vi "Signals.Scale.Raw.vi"(6 "Type":T1, 7 "Lookup":variant, 8 "error in":errorcluster, 10 "ID":u32, 11 "Writes Ref":T2) -> (0 "error out":errorcluster, 2 "Data":u8[](array[numeric]))   [LabVIEW 2019, in "Diagnostics Addon Engine.lvlib"]
uses:
  Diagnostics Addon Engine.lvlib
  <vilib>/NI/NIVS Inline Async API/_Data Access Engine/Data Access Engine/Types/Read.DVR.ctl
  <vilib>/NI/NIVS Inline Async API/_Data Access Engine/Access Type Classes/Read/Read.lvclass
  Shared/Types/Type.ctl
  Shared/Types/Frame.Lookup.Info.ctl
  <vilib>/NI/NIVS Inline Async API/_Data Access Engine/Access Type Classes/Read/Read.lvclass/Read.ctl
  <vilib>/NI/NIVS Inline Async API/_Data Access Engine/Data Access Engine/Methods/Read.Data.vi
  <vilib>/NI/NIVS Inline Async API/_Data Access Engine/Access Type Classes/Read/Read.ProcessData.vi
  Shared/SubVIs/Constants.vi
  <vilib>/xnet/xnet.llb/XNET Convert (Signal to Frame CAN).vi
  Shared/Diagnostics Addon Shared.lvlib
  <vilib>/NI VeriStand/Custom Device Tools/Custom Device Utility Library/Custom Device Utility Library.lvlib
  <vilib>/NI/NIVS Inline Async API/_Data Access Engine/Data Access Engine/Data Access Engine.lvclass
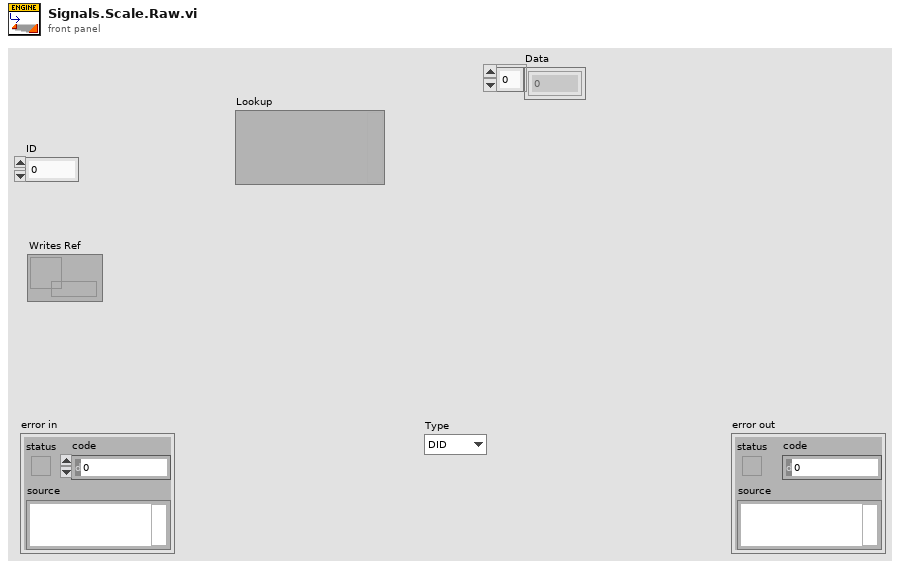
[diagram p1: front panel]
types:
  T1 = typedef "Diagnostics Addon Shared.lvlib/Type.ctl" = enum16{"DID", "CDID", "PID", "CPID", "Read Memory", "Write Memory", "DTC Control", "IO Cmd", "IO Resp", "Routine Start Cmd", "Routine Start Resp", "Routine Request Cmd", "Routine Request Resp", "Routine Stop Cmd", "Routine Stop Resp", "UserDefined Cmd", "UserDefined Rsp"}
  T2 = typedef "Data Access Engine.lvlib/Data Access Engine.lvclass/Read.DVR.ctl" = refnum<data-value>
  T3 = typedef "Diagnostics Addon Shared.lvlib/Frame.Lookup.Info.ctl" = cluster{"Offset":i32, "Length":i32, "ByteLength":u16}
  T4 = typedef "XNET Frame CAN.ctl" = cluster{"timestamp":timestamp, "payload":u8[], "identifier":u32, "type":T5, "extended?":bool, "echo?":bool}
  T5 = typedef "XNET Frame Type CAN.ctl" = u8
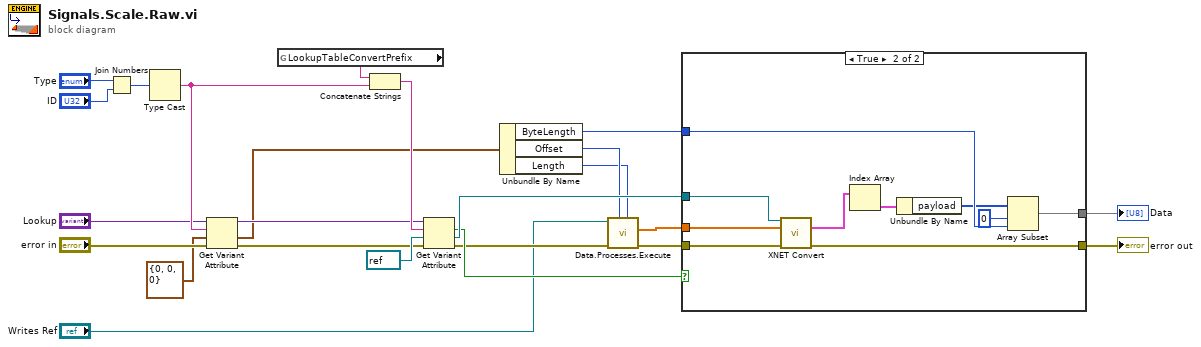
[diagram p0: block diagram]
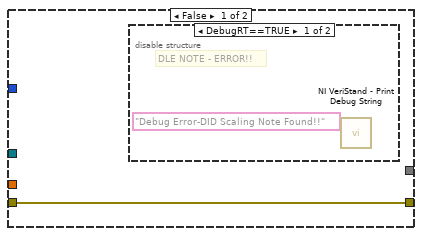
[diagram p2: hidden frame]
diagram:
  n1 = Join Numbers(hi="Type", lo="ID") -> ((hi.lo)=w8:u64)
  n2 = Type Cast(x=w8) -> (*(type *) &x=w18:string)  [unwired: 1 in]
  n3 = Get Variant Attribute(Variant="Lookup", name=w18, default value (empty Variant)=T3 {"Offset"=0, "Length"=0, "ByteLength"=0} ("cluster"), error in="error in") -> (duplicate Variant=w17:variant, value=w12:T3, error out=w19:errorcluster)  [unwired: 1 out]
  n4 = global read "Constants.vi" "LookupTableConvertPrefix"() -> (w20:string)
  n5 = Concatenate Strings(w20, w18) -> (w21:string)
  n6 = Get Variant Attribute(Variant=w17, name=w21, default value (empty Variant)=refnum<k21> refnum ("DID Conversion"), error in=w19) -> (found=w7:bool, value=w13:refnum<k21>, error out=w3:errorcluster)  [unwired: 1 out]
  n7 = Unbundle By Name(w12) -> ("ByteLength"=w15:u16, "Offset"=w6:i32, "Length"=w5:i32)
  n8 = call-poly <vilib>:"Data.Processes.Execute.vi"("length"=w5, "index"=w6, "error in (no error)"=w3, "Ref"="Writes Ref") -> ("error out"=w2:errorcluster, "Values"=w4:dbl[])  [unwired: 5 in, 1 out]
  n9 = case shown="True" w7 {
    tunnel: w2 -> [w25 w36]
    tunnel: [w25 w30] -> w11
    tunnel: w4 -> [_ w32]
    tunnel: w13 -> [_ w35]
    tunnel: w15 -> [_ w33]
    tunnel: [_ w31] -> w14
    frame False {
      n10 = disable-structure shown="DebugRT==TRUE" {
        frame condition #0 {
          # "DLE NOTE - ERROR!!"
          n11 = call <vilib>:"NI VeriStand - Print Debug String.vi"("Message"="Debug Error-DID Scaling Note Found!!" ("Debug String")) -> ()  [unwired: 10 in, 1 out]
        }
        frame condition #1 (active) {
        }
      }
    }
    frame True {
      n12 = call-poly <vilib>:"XNET Convert.vi"("session in"=w35, "signal data"=w32, "error in (no error)"=w36) -> ("frame data"=w29:T4[], "error out"=w30:errorcluster)  [unwired: 9 in, 2 out]
      n13 = Index Array(array=w29) -> (element=w28:T4)  [unwired: 1 in]
      n14 = Unbundle By Name(w28) -> ("payload"=w27:u8[])
      n15 = Array Subset(array=w27, index=0, length=w33) -> (w31:u8[])
    }
  }
  "error out" <- w11
  "Data" <- w14
